vi "ConfigAuthenticationTimeout.vi"(7 "timer function":T1, 8 "error in (no error)":errorcluster, 10 "reconnect in":T2={"ReconnectInterval"=0.0, "BaseReconnectInterval"=0.0, "AuthAttempts"=0, "MaxAttempts"=10}, 11 "Qbus in":refnum<class "Qbus.lvclass">) -> (0 "error out":errorcluster, 2 "reconnect out":T2={"ReconnectInterval"=0.0, "BaseReconnectInterval"=0.0, "AuthAttempts"=0, "MaxAttempts"=10}, 3 "Qbus out":refnum<class "Qbus.lvclass">)   [LabVIEW 2017, in "ServerComm.lvlib"]
uses:
  <vilib>/addons/InsightCM/Devices/Shared/Common/ServerComm/ServerComm.lvlib
  <vilib>/addons/InsightCM/Devices/Shared/Common/ServerComm/controls/ReconnectData.ctl
  <vilib>/addons/Qbus/Qbus.lvclass
  <vilib>/addons/InsightCM/Devices/Shared/Common/ServerComm/controls/TimerFunction.ctl
  <vilib>/addons/TimerProcess/controls/taskType.ctl
  <vilib>/addons/TimerProcess/TimerProcess.lvlib
  <vilib>/addons/TraceLogger/TraceLogger.lvlib
  <vilib>/addons/InsightCM/Devices/Shared/Common/Controller/Controller.lvlib
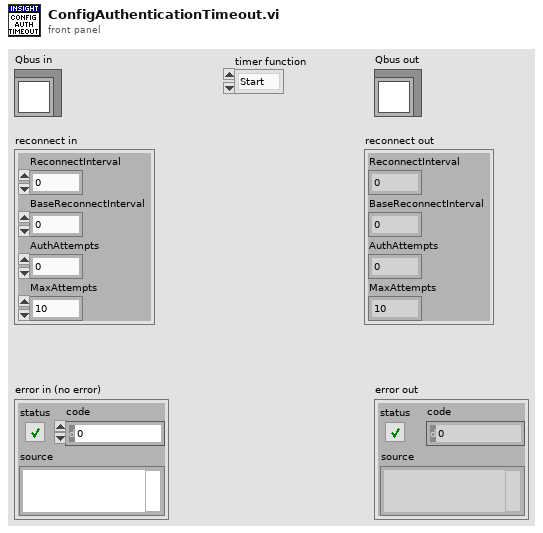
[diagram p1: front panel]
types:
  T1 = typedef "ServerComm.lvlib/TimerFunction.ctl" = enum16{"Start", "Stop", "Reset"}
  T2 = typedef "ServerComm.lvlib/ReconnectData.ctl" = cluster{"ReconnectInterval":dbl, "BaseReconnectInterval":dbl, "AuthAttempts":i32, "MaxAttempts":i32}
  T3 = typedef "TimerProcess.lvlib/taskType.ctl" = enum16{"single", "repeat"}
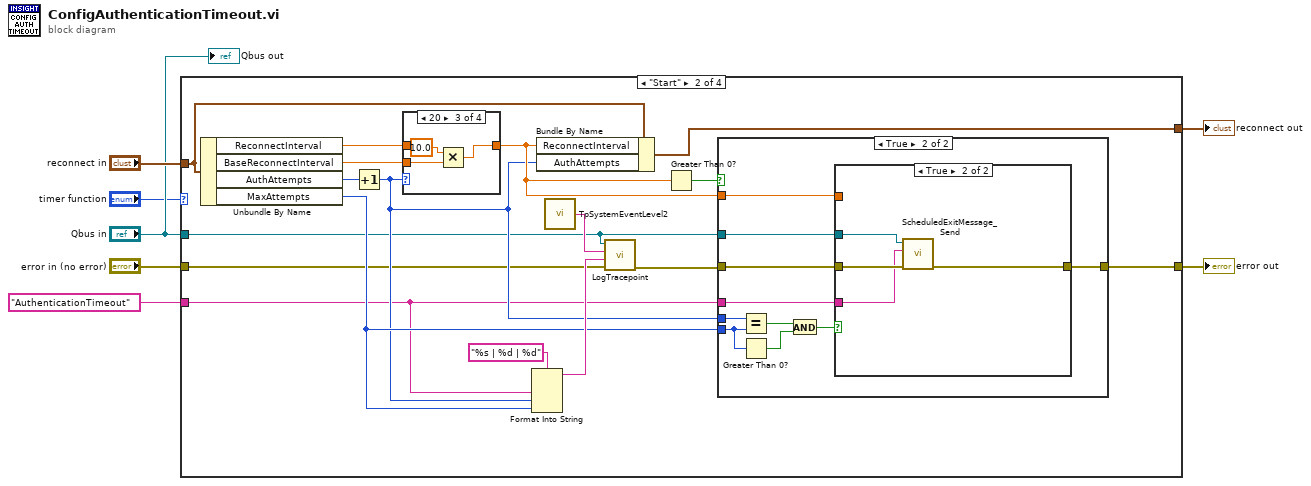
[diagram p0: block diagram]
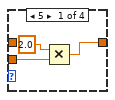
[diagram p3: hidden frame]
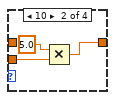
[diagram p4: hidden frame]
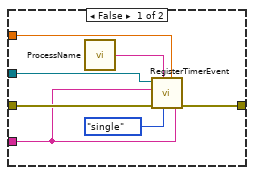
[diagram p7: hidden frame]
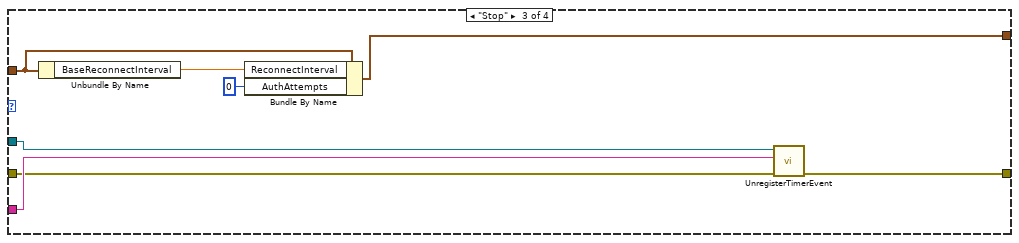
[diagram p8: hidden frame]
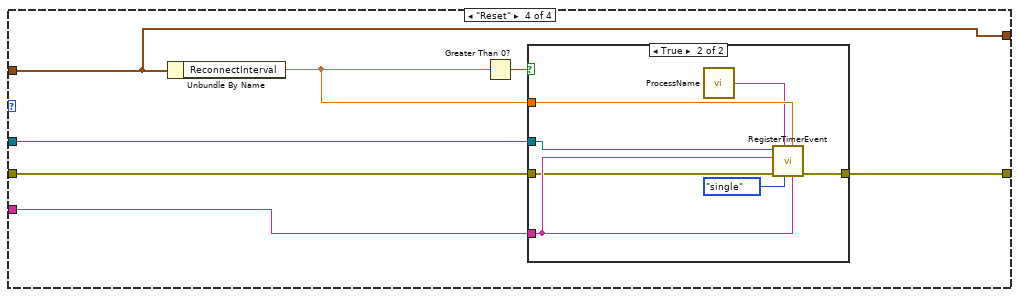
[diagram p9: hidden frame]
diagram:
  n1 = case shown="\"Start\"" "timer function" {
    tunnel: "reconnect in" -> [w8 w22 w62 w67]
    tunnel: "Qbus in" -> [_ w10 w66 w69]
    tunnel: "AuthenticationTimeout" ("CallBackAction") -> [_ w13 w65 w68]
    tunnel: "error in (no error)" -> [w9 w12 w64 w71]
    tunnel: [w9 w26 w63 w72] -> w5
    tunnel: [w8 w20 w59 w67] -> w2
    frame Default {
    }
    frame "Start" {
      n2 = Unbundle By Name(w22) -> ("ReconnectInterval"=w23:dbl, "BaseReconnectInterval"=w24:dbl, "AuthAttempts"=w19:i32, "MaxAttempts"=w15:i32)
      n3 = Increment(x=w19) -> (x+1=w14:i32)
      n4 = case shown="20" w14 {
        tunnel: w24 -> [w28 w31 w34 _]
        tunnel: w23 -> [_ _ _ w36]
        tunnel: [w29 w32 w35 w36] -> w21
        frame 5 {
          n5 = Multiply(x=2.0, y=w28) -> (x*y=w29:dbl)
        }
        frame 10 {
          n6 = Multiply(x=5.0, y=w31) -> (x*y=w32:dbl)
        }
        frame 20 {
          n7 = Multiply(x=10.0, y=w34) -> (x*y=w35:dbl)
        }
        frame Default {
        }
      }
      n8 = Format Into String(format string="%s | %d | %d", w13, w14, w15) -> (resulting string=w18:string)  [unwired: 2 in, 1 out]
      n9 = Bundle By Name(cluster=w22, "ReconnectInterval"=w21, "AuthAttempts"=w14) -> (w20:T2)
      n10 = call <vilib>:"TpSystemEventLevel2.vi"() -> ("tracepoint name"=w17:string)  [unwired: 5 in]
      n11 = call <vilib>:"LogTracepoint.vi"("error in (no error)"=w12, "log string"=w18, "tracepoint"=w17, "qbus in"=w10) -> ("error out"=w11:errorcluster)  [unwired: 6 in, 1 out]
      n12 = Greater Than 0?(x=w21) -> (x > 0?=w25:bool)
      n13 = case shown="True" w25 {
        tunnel: w21 -> [_ w44]
        tunnel: w10 -> [_ w43]
        tunnel: w13 -> [_ w45]
        tunnel: w11 -> [w37 w47]
        tunnel: [w37 w46] -> w26
        tunnel: w14 -> [_ w42]
        tunnel: w15 -> [_ w41]
        frame False {
        }
        frame True {
          n14 = Equal?(x=w42, y=w41) -> (x = y?=w39:bool)
          n15 = Greater Than 0?(x=w41) -> (x > 0?=w40:bool)
          n16 = And(x=w39, y=w40) -> (x .and. y?=w38:bool)
          n17 = case shown="True" w38 {
            tunnel: w47 -> [w50 w57]
            tunnel: [w53 w58] -> w46
            tunnel: w45 -> [w49 w55]
            tunnel: w44 -> [w52 _]
            tunnel: w43 -> [w51 w56]
            frame False {
              n18 = call <vilib>:"ProcessName.vi"() -> ("process name"=w48:string)  [unwired: 5 in]
              n19 = call <vilib>:"RegisterTimerEvent.vi"("timer task name"=w49, "interval (sec)"=w52, "type"=taskType."single", "process name"=w48, "error in (no error)"=w50, "callback action"=w49, "qbus in"=w51) -> ("error out"=w53:errorcluster)  [unwired: 3 in, 1 out]
            }
            frame True {
              n20 = call <vilib>:"ScheduledExitMessage_Send.vi"("error in (no error)"=w57, "scheduled exit reason"=w55, "Qbus in"=w56) -> ("error out"=w58:errorcluster)  [unwired: 7 in, 1 out]
            }
          }
        }
      }
    }
    frame "Stop" {
      n21 = Unbundle By Name(w62) -> ("BaseReconnectInterval"=w61:dbl)
      n22 = Bundle By Name(cluster=w62, "ReconnectInterval"=w61, "AuthAttempts"=0) -> (w59:T2)
      n23 = call <vilib>:"UnregisterTimerEvent.vi"("error in (no error)"=w64, "timer task name"=w65, "qbus in"=w66) -> ("error out"=w63:errorcluster)  [unwired: 7 in, 1 out]
    }
    frame "Reset" {
      n24 = Unbundle By Name(w67) -> ("ReconnectInterval"=w70:dbl)
      n25 = Greater Than 0?(x=w70) -> (x > 0?=w73:bool)
      n26 = case shown="True" w73 {
        tunnel: w70 -> [_ w81]
        tunnel: w69 -> [_ w80]
        tunnel: w68 -> [_ w79]
        tunnel: w71 -> [w74 w76]
        tunnel: [w74 w75] -> w72
        frame False {
        }
        frame True {
          n27 = call <vilib>:"ProcessName.vi"() -> ("process name"=w78:string)  [unwired: 5 in]
          n28 = call <vilib>:"RegisterTimerEvent.vi"("timer task name"=w79, "interval (sec)"=w81, "type"=taskType."single", "process name"=w78, "error in (no error)"=w76, "callback action"=w79, "qbus in"=w80) -> ("error out"=w75:errorcluster)  [unwired: 3 in, 1 out]
        }
      }
    }
  }
  "error out" <- w5
  "reconnect out" <- w2
  "Qbus out" <- "Qbus in"
